vi "get_just1_analog.vi"() -> ()   [LabVIEW 2018]
uses:
  <vilib>/rvi/Emulation/niFpgaGetClockAttributes.vi
  <vilib>/rvi/Emulation/niFpgaSctlEmulationGetInTimedLoop.vi
  <vilib>/rvi/Emulation/niFpgaEmulationReportErrorSimple.vi
  <vilib>/rvi/eio/common/nirviEmuTemplateMethod_errors.vi
  <vilib>/rvi/Emulation/niFpgaCriticalErrorInLSC.vi
  <vilib>/eio/EIONode/EIONode.xnode
panel:
  out "32bit integer":i32
  out "Mod1/AI14":fxp<+/-,24,5>
  in  "stop":bool
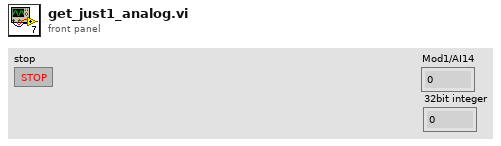
[diagram p1: front panel]
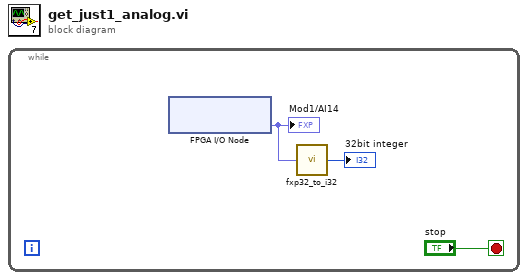
[diagram p0: block diagram]
diagram:
  n1 = while {
    stop <- "stop" stop-if-true
    n2 = xnode "FPGA I/O Node"() -> ("Mod1/AI14"=w2:fxp<+/-,24,5>)  [unwired: 1 in, 1 out]
    "Mod1/AI14" <- w2
    n3 = call "fxp32_to_i32.vi"("fxp32_16"=w2) -> ("32bit integer"=→"32bit integer":i32)
  }
